vi "AFG3352X.use external amplitude modulation.vi"(0 "i ref in":refnum<vi>, 3 "ms timeout (10000)":i32=10000, 5 "error in (no error)":errorcluster) -> (14 "i ref out":refnum<vi>, 17 "timed out":bool, 19 "error out":errorcluster)   [LabVIEW 2014, in "AFG3352X.lvlib"]
doc: "Enables external amplitude modulation of the device."
uses:
  AFG3352X.lvlib
  CSCore/CSApplicationBaseClasses/AFGBase/AFGBase.serviceType.ctl
  CSCore/CSApplicationBaseClasses/AFGBase/AFGBase.directionType.ctl
  CSlibraries/UtilityLib/UtilityLib.valueStatus.ctl
  CSCore/CSApplicationBaseClasses/AFGBase/AFGBase.waveformType.ctl
  CSCore/CSApplicationBaseClasses/DeviceBase/DeviceBase.lvlib
  CSCore/CSApplicationBaseClasses/AFGBase/AFGBase.lvlib
  CSlibraries/UtilityLib/UtilityLib.lvlib
  CSinstr.lib/Agilent 3352X Series/Agilent 3352X Series.lvlib
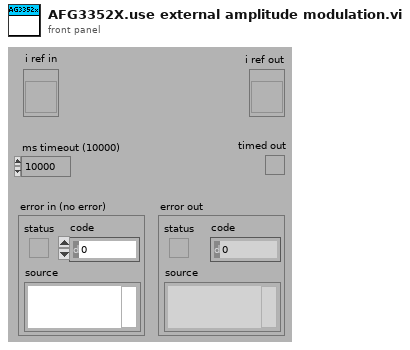
[diagram p1: front panel]
types:
  T1 = typedef "AFGBase.lvlib/AFGBase.waveformType.ctl" = enum16{"sine", "square", "ramp", "pulse", "noise", "DC", "arbitrary", "triangle", "ramp_up", "ramp_down", "amplitude modulation"}
  T2 = typedef "UtilityLib.lvlib/UtilityLib.valueStatus.ctl" = enum16{"no info available", "stand by/off", "on", "warning", "alarm/malfunction", "not implemented", "user action required", "important information", "system default", "control default", "indicator default", "button default"}
  T3 = typedef "AFGBase.lvlib/AFGBase.directionType.ctl" = enum16{"unknown", "update actual value", "update nominal value", "update both"}
  T4 = typedef "AFGBase.lvlib/AFGBase.serviceType.ctl" = enum16{"frequency", "amplitude", "phase", "DCOffset", "enableOutput", "trigger", "waveformType"}
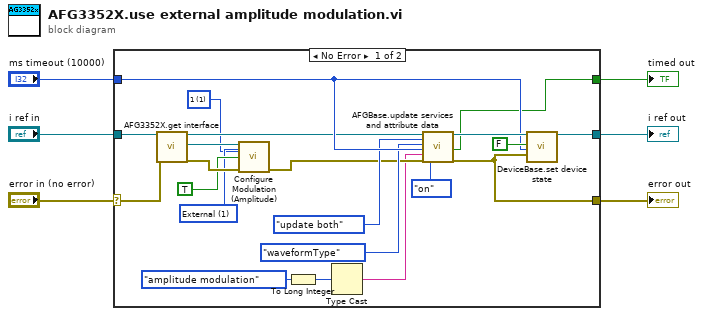
[diagram p0: block diagram]
diagram:
  n1 = case shown="No Error" "error in (no error)" {
    selector: "error in (no error)" -> [w18 w28]
    tunnel: [w27 w29] -> w6
    tunnel: "ms timeout (10000)" -> [w23 _]
    tunnel: "i ref in" -> [w19 w29]
    tunnel: [w24 w28] -> w2
    tunnel: [w8 _] -> w1
    frame No Error {
      w7 = 1 items=["1"=1, "2"=2] ("Channel (1: 1)")
      w12 = 1 items=["Internal", "External"] ("AM Source (0: Internal)")
      n2 = call "AFG3352X.get interface.vi"("i ref in"=w19, "error in (no error)"=w18) -> ("i ref out"=w17:refnum<vi>, "interface"=w15:refnum<visa-resource-name>, "error out"=w16:errorcluster)  [unwired: 15 in]
      n3 = call "Configure Modulation (Amplitude).vi"("VISA resource name"=w15, "AM Source (0: Internal)"=w12, "Channel (1: 1)"=w7, "Enable AM (T: Enable)"=TRUE ("Enable Amplitude Modulation (True)"), "error in (no error)"=w16) -> ("error out"=w14:errorcluster)  [unwired: 9 in, 1 out]
      n4 = To Long Integer(number=AFGBase.waveformType."amplitude modulation" ("waveformType")) -> (32bit integer=w9:i32)
      n5 = Type Cast(x=w9) -> (*(type *) &x=w11:string)  [unwired: 1 in]
      n6 = call "AFGBase.update services and attribute data.vi"("i ref in"=w17, "direction"=AFGBase.directionType."update both", "service"=AFGBase.serviceType."waveformType", "ms timeout (10000)"=w23, "value"=w11, "error in (no error)"=w14, "quality"=UtilityLib.valueStatus."on") -> ("i ref out"=w25:refnum<vi>, "timed out"=w8:bool, "error out"=w24:errorcluster)  [unwired: 10 in]
      n7 = call "DeviceBase.set device state.vi"("i ref in"=w25, "implicit"=FALSE, "ms timeout (10000)"=w23, "device error"=w24) -> ("i ref out"=w27:refnum<vi>)  [unwired: 13 in, 2 out]
    }
    frame Error {
    }
  }
  "error out" <- w2
  "i ref out" <- w6
  "timed out" <- w1
